vi "Read String.vi"(7 "section":string, 8 "error in":errorcluster, 9 "default":string, 10 "key":string, 11 "config file in":refnum<data-value>) -> (0 "error out":errorcluster, 1 "value":string, 2 "found?":bool, 3 "config file out":refnum<data-value>)   [LabVIEW 2012, in "configlib.lvlib"]
uses:
  configlib.lvlib
  Configuration File Definition.ctl
  File Options.ctl
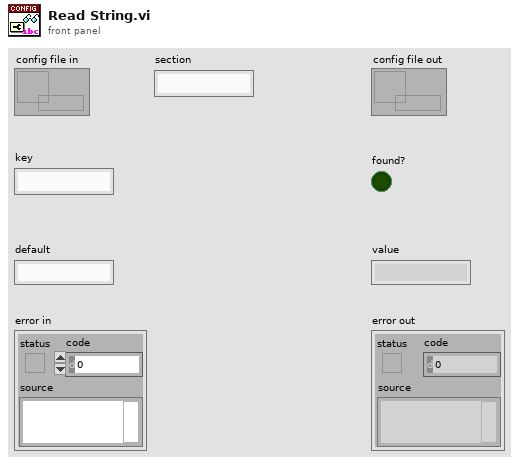
[diagram p1: front panel]
types:
  T1 = typedef "configlib.lvlib/Configuration File Definition.ctl" = cluster{"dirty":bool, "path":path, "Fileopts":T2, "Section Lookup":variant, "Key Lookup":variant, "Raw File":string[]}
  T2 = typedef "configlib.lvlib/File Options.ctl" = cluster{"Name/Value delimiter (\"=\")":string, "Comment delimiter (\";\")":string}
  T3 = typedef "configlib.lvlib/Key Definition.ctl" = cluster{"Line Number":i32, "Value":string}
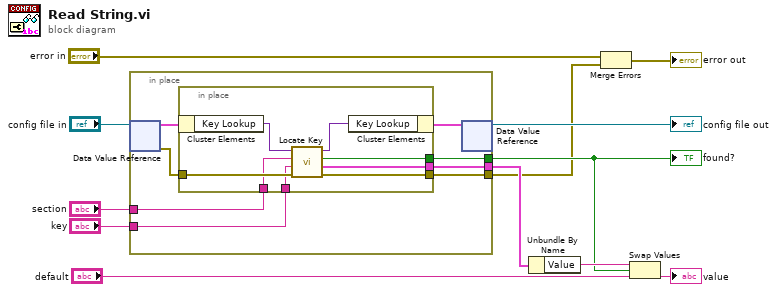
[diagram p0: block diagram]
diagram:
  n1 = in-place {
    in-place-border: "key" -> [w14]
    in-place-border: "section" -> [w13]
    in-place-border: [w17] -> w3
    in-place-border: [w16] -> w9
    in-place-border: [w15] -> w5
    n2 = in-place-dvr #1("config file in") -> (w20:T1, w18:errorcluster)
    n3 = in-place {
      in-place-border: w18 -> [w26]
      in-place-border: [w25] -> w17
      in-place-border: [w24] -> w16
      in-place-border: [w23] -> w15
      in-place-border: w14 -> [w22]
      in-place-border: w13 -> [w21]
      n4 = in-place-cluster #2(w20) -> ("Key Lookup"=w28:variant)
      n5 = call "Locate Key.vi"("error in"=w26, "key"=w22, "section"=w21, "key lookup"=w28) -> ("error out"=w25:errorcluster, "key definition"=w24:T3, "found?"=w23:bool, "key lookup out"=w27:variant)  [unwired: 4 in]
      n6 = in-place-cluster #2("Key Lookup"=w27) -> (w19:T1)
    }
    n7 = in-place-dvr #1(w19) -> (→"config file out":refnum<data-value>)  [unwired: 1 out]
  }
  "found?" <- w5
  n8 = Unbundle By Name(w9) -> ("Value"=w8:string)
  n9 = Merge Errors("error in", w3) -> (→"error out":errorcluster)
  n10 = Swap Values(12:w8, 13:w5, 14:"default") -> (3:→"value":string)  [unwired: 1 out]
